vi "TypeDescriptor_GetType.vi"(11 "type descriptor":i16[](array[numeric])) -> (2 "Type":u8 format="%.0x", 3 "type descriptor dup":i16[](array[numeric]))   [LabVIEW 2013, in "OpenDescriptor.lvlib"]
uses:
  OpenDescriptor.lvlib
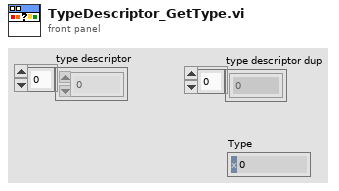
[diagram p1: front panel]
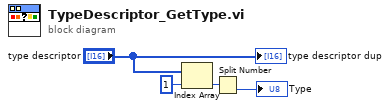
[diagram p0: block diagram]
diagram:
  n1 = Index Array(array="type descriptor", index=1) -> (element=w4:i16)
  n2 = Split Number(x=w4) -> (lo(x)=→"Type":u8)  [unwired: 1 out]
  "type descriptor dup" <- "type descriptor"
